vi "Insulation Resistance Results Parse.vi"(8 "error in (no error)":errorcluster, 10 "Insulation Resistance Results In":string[](array[string])) -> (0 "error out":errorcluster, 2 "Insulation Resistance":string)   [LabVIEW 2018]
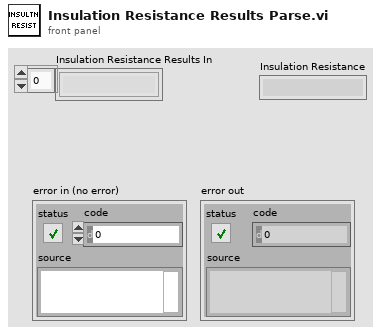
[diagram p1: front panel]
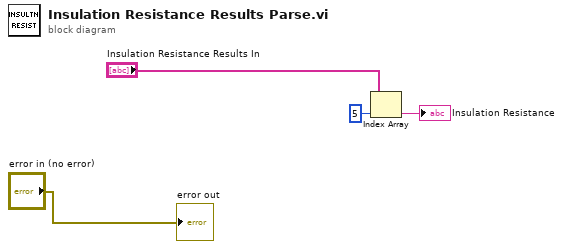
[diagram p0: block diagram]
diagram:
  n1 = Index Array(array="Insulation Resistance Results In", index=5) -> (element=→"Insulation Resistance":string)
  "error out" <- "error in (no error)"
